vi "On Success.vi"(8 "error in (no error)":errorcluster, 9 "Session In":refnum<class "Session.lvclass">, 10 "User":refnum<class "User.lvclass">, 11 "FormAuthentication in":refnum<class "FormAuthentication.lvclass">) -> (0 "error out":errorcluster, 1 "Session":refnum<class "Session.lvclass">, 2 "Response":refnum<class "Response.lvclass">, 3 "FormAuthentication out":refnum<class "FormAuthentication.lvclass">)   [LabVIEW 2020, in "HTTP Server.lvlib" / "FormAuthentication.lvclass"]
uses:
  FormAuthentication.lvclass
  <vilib>/IlluminatedG/IG HTTP Utils/HTTP Utils/Response/Response.lvclass
  Session/Session.lvclass
  User/User.lvclass
  Redirect Response/Redirect Response.lvclass
  C:/Program Files (x86)/National Instruments/LabVIEW 2020/vi.lib/IlluminatedG/IG HTTP Utils/HTTP Utils/Response/Response.lvclass
  FormAuthentication.lvclass/FormAuthentication.ctl
  <vilib>/IlluminatedG/lv-stream/URI/URI.lvclass
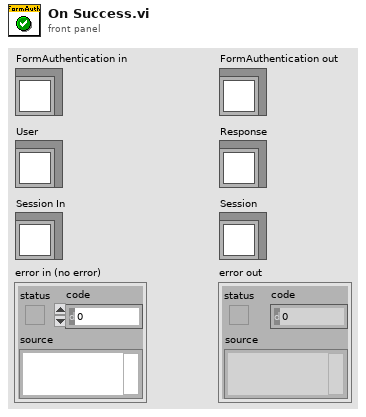
[diagram p1: front panel]
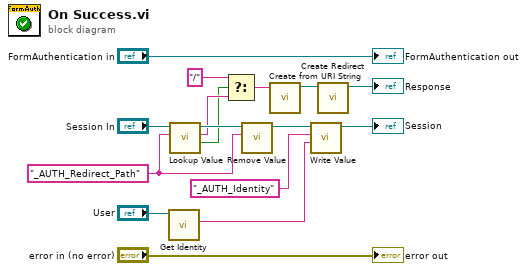
[diagram p0: block diagram]
diagram:
  w12 = "_AUTH_Redirect_Path" ("Name")
  n1 = call-dynamic "Get Identity.vi"("User in"="User") -> ("Identity"=w1:string)  [unwired: 8 in, 2 out]
  n2 = call "Lookup Value.vi"("Name"=w12, "Session in"="Session In") -> ("Not Found?"=w10:bool, "Value"=w11:string, "Session out"=w13:refnum<class "Session.lvclass">)  [unwired: 6 in, 1 out]
  n3 = Select(t="/", s=w10, f=w11) -> (s? t:f=w8:string)
  n4 = call "Remove Value.vi"("Name"=w12, "Session in"=w13) -> ("Session out"=w4:refnum<class "Session.lvclass">)  [unwired: 6 in, 3 out]
  n5 = call <vilib>:"Create from URI String.vi"("URI String"=w8) -> ("URI out"=w7:refnum<class "URI.lvclass">)  [unwired: 9 in, 1 out]
  n6 = call "Write Value.vi"("Value"=w1, "Name"="_AUTH_Identity", "Session in"=w4) -> ("Session out"=→"Session":refnum<class "Session.lvclass">)  [unwired: 6 in, 2 out]
  n7 = call "Create Redirect.vi"("Redirect URI"=w7) -> ("Redirect Response out"=→"Response":refnum<class "Redirect Response.lvclass">)  [unwired: 9 in, 1 out]
  "error out" <- "error in (no error)"
  "FormAuthentication out" <- "FormAuthentication in"
